vi "Robot Global Data.vi"() -> ()   [LabVIEW 2023]
doc: "This global VI can contain as many global variables as you need. To create a global variable, place a control on the panel, give it a good name. To read or write to it from a VI, drag the icon to the diagram of that VI. You can also drag from the project. Click on the node to change which global you access. You shouldn't have multiple locations writing to a global or it will cause a race-condition."
uses:
  <vilib>/Rock Robotics/WPI/Camera/WPI_CameraImageSize.ctl
  <vilib>/Rock Robotics/WPI/DriverStation/WPI_DriverStationRobotMode2.ctl
panel:
  out "Distance to AT":dbl
  in  "Length":dbl
  in  "Width":dbl
  in  "GameCube?":bool
  in  "LED STATE":enum16{"NORMAL", "RAINBOW"}(ring)
  in  "Lower Arm Offset":dbl
  in  "Upper Arm Offset":dbl
  out "Arm set":bool=TRUE
  in  "Lower Arm Encoder Goal":dbl=271.0227272727273
  in  "Upper Arm Encoder Goal":dbl=341.3352272727273
  in  "Current Game Piece":enum16{"Cone", "Cube", "None"}(ring)=enum."None"
  in  "Grabber State":enum16{"Closed", "Open"}(ring)
  in  "Inatke Out":bool
  in  "Arm Position":T1(ring)=enum."Transfer"
  out "Detected Tags":T2(array[cluster])
  in  "target":T3(ring)=enum."Cube"
  out "VisionAngle":dbl
  out "Result":T4 {"Score" format="%#_3g"; "Pixels"."Rectangle"."Numeric 5" format="%#_3g"; "Pixels"."Rectangle"."Numeric 3" format="%#_3g"; "Pixels"."Rectangle"."Numeric 2" format="%#_3g"; "Pixels"."Rectangle"."Numeric" format="%#_3g"; "Normalized"."Rectangle"."Numeric 5" format="%#_2g"; "Normalized"."Rectangle"."Numeric 3" format="%#_2g"; "Normalized"."Rectangle"."Numeric 2" format="%#_2g"; "Normalized"."Rectangle"."Numeric" format="%#_2g"; "Normalized"."Center"."?" format="%#_3g"; "Normalized"."Center"."?" format="%#_3g"; "Distance (ft)" format="%#_3g"}
  in  "Robot Mode":T5=enum."Finish"
  in  "image size":T6=enum."320x240"
  in  "Enable Vision":bool
  # "Legnth and Width from\nbottom of each wheel"
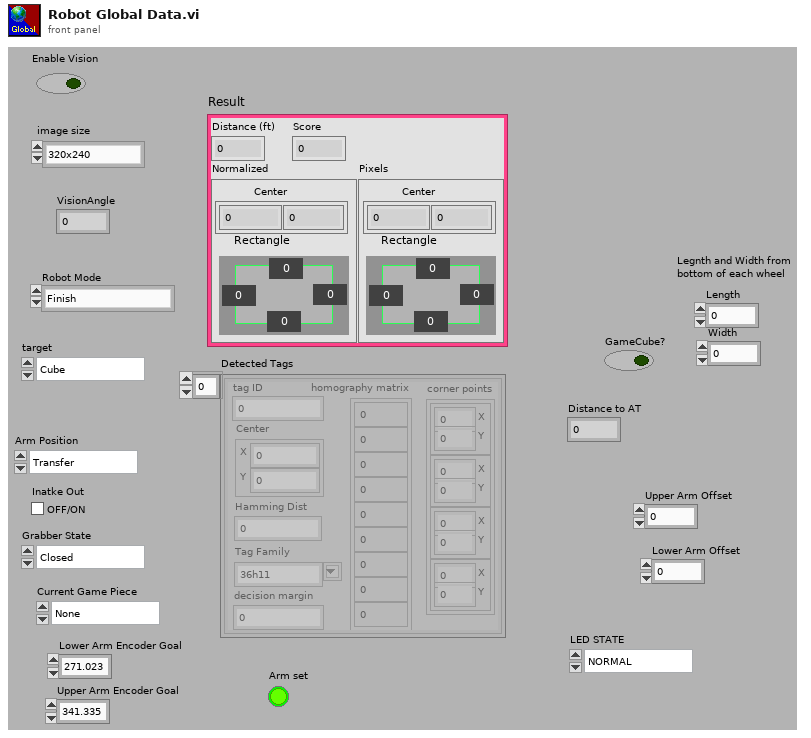
[diagram p1: front panel]
types:
  T1 = enum16{"Station?", "Transfer", "Node 2", "Node 1", "Node 0"}
  T2 = cluster{"tag ID":i32, "Center":cluster{"X":dbl, "Y":dbl}, "homography matrix":dbl[], "decision margin":dbl, "Hamming Dist":i32, "corner points":cluster{"X":dbl, "Y":dbl}[], "Tag Family":string}[]
  T3 = enum16{"AprilTag", "Reflective Tape", "Custom", "Cube", "Cone"}
  T4 = cluster{"Distance (ft)":dbl, "Score":dbl, "Normalized":cluster{"Center":cluster{dbl, dbl}, "Rectangle":cluster{"Numeric":dbl, "Numeric 2":dbl, "Numeric 3":dbl, "Numeric 5":dbl}}, "Pixels":cluster{"Center":cluster{dbl, dbl}, "Rectangle":cluster{"Numeric":dbl, "Numeric 2":dbl, "Numeric 3":dbl, "Numeric 5":dbl}}}
  T5 = typedef "WPI_DriverStationRobotMode2.ctl" = enum16{"Autonomous Disabled", "Autonomous Enabled", "Teleop Disabled", "Teleop Enabled", "Disconnected", "Finish", "Test Disabled", "Test Enabled", "Emergency Stopped"}
  T6 = typedef "WPI_CameraImageSize.ctl" = enum16{"640x480", "320x240", "160x120", "Custom"}
diagram:
